vi "Numric.vi"(7 "x":dbl, 11 "y":dbl) -> (8 "x = y?":bool)   [LabVIEW 2015]
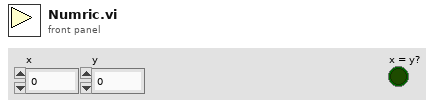
[diagram p1: front panel]
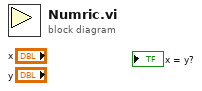
[diagram p0: block diagram]
diagram:
